vi "RunCaller.vi"(8 "error in (no error)":errorcluster, 11 "BaseDriver in":refnum<class "BaseDriver.lvclass">) -> (0 "error out":errorcluster, 3 "BaseDriver out":refnum<class "BaseDriver.lvclass">)   [LabVIEW 2013, in "BaseDriver.lvclass"]
doc: "This Vi simply calls the dynamic dispatch method Run. It exists purely so that there is a way to call Run using start asynchronous call"
uses:
  BaseDriver.lvclass
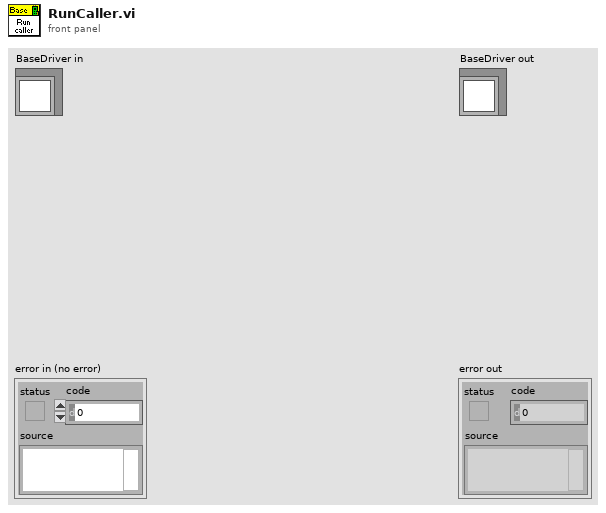
[diagram p1: front panel]
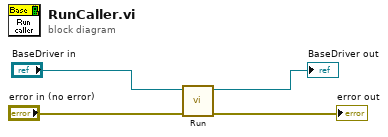
[diagram p0: block diagram]
diagram:
  n1 = call-dynamic "Run.vi"("error in (no error)"="error in (no error)", "BaseDriver in"="BaseDriver in") -> ("error out"=→"error out":errorcluster, "BaseDriver out"=→"BaseDriver out":refnum<class "BaseDriver.lvclass">)  [unwired: 8 in]
